vi "CaculateIntControl.vi"(10 "stringControl":refnum<vi> caption="컨트롤 참조 번호", 11 "category":enum16{"add", "minus"}(ring)) -> ()   [LabVIEW 2018]
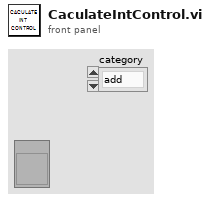
[diagram p1: front panel]
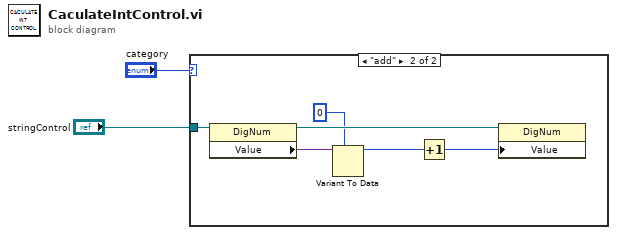
[diagram p0: block diagram]
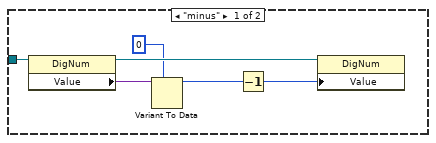
[diagram p2: hidden frame]
diagram:
  n1 = case shown="\"add\"" "category" {
    tunnel: "stringControl" -> [w8 w14]
    frame "minus" {
      n2 = property class="DigNum"(reference=w8) -> (reference out=w7:refnum<vi>, "Value"=w6:variant)  [unwired: 1 in, 1 out]
      n3 = Variant To Data(type=0, Variant=w6) -> (data=w4:i32)  [unwired: 1 in, 1 out]
      n4 = Decrement(x=w4) -> (x-1=w3:i32)
      n5 = property class="DigNum"(reference=w7, "Value"=w3) -> ()  [unwired: 1 in, 2 out]
    }
    frame "add" {
      n6 = property class="DigNum"(reference=w14) -> (reference out=w13:refnum<vi>, "Value"=w12:variant)  [unwired: 1 in, 1 out]
      n7 = Variant To Data(type=0, Variant=w12) -> (data=w10:i32)  [unwired: 1 in, 1 out]
      n8 = Increment(x=w10) -> (x+1=w9:i32)
      n9 = property class="DigNum"(reference=w13, "Value"=w9) -> ()  [unwired: 1 in, 2 out]
    }
  }
